vi "Store Static VI References for Subpanel.vi"(8 "error in (no error)":errorcluster, 11 "Controller Configuration in":refnum<class "Controller Configuration.lvclass">) -> (0 "error out":errorcluster, 3 "Controller Configuration out":refnum<class "Controller Configuration.lvclass">)   [LabVIEW 2016, in "Msmt Configuration.lvlib" / "Controller Configuration.lvclass"]
uses:
  Controller Configuration.lvclass
  \\Mac\Home/Documents/Extensible-Config-Dialog/Configuration.lvclass
  Extensible-Config-Dialog/Configuration.lvclass
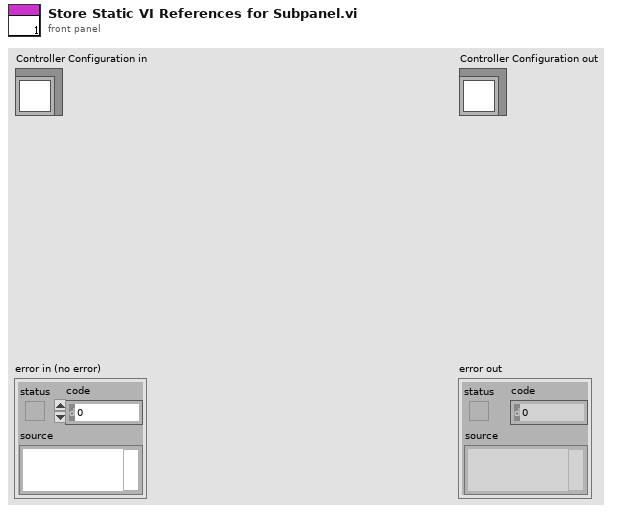
[diagram p1: front panel]
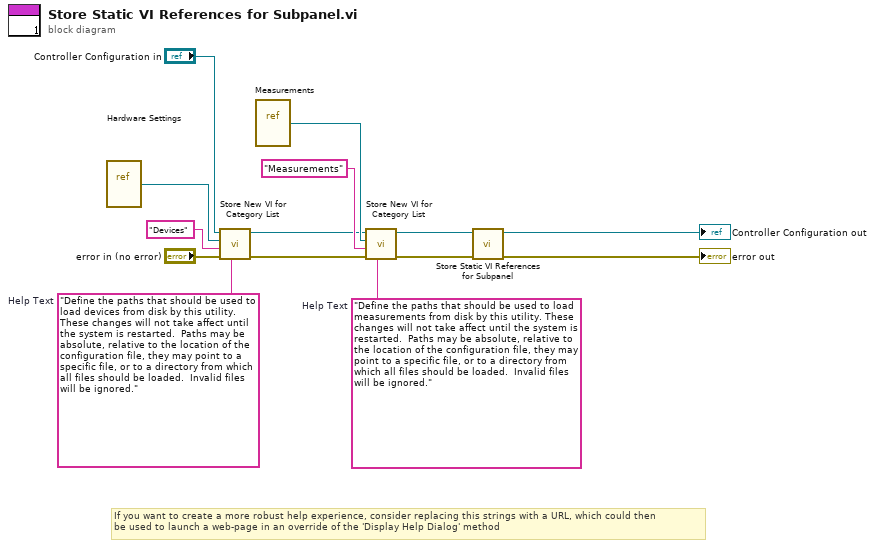
[diagram p0: block diagram]
diagram:
  w1 = "Define the paths that should be used to load devices from disk by this utility. These changes will not take affect until the system is restarted.  Paths may be absolute, relative to the location of the configuration file, they may point to a specific file, or to a directory from which all files should be loaded.  Invalid files will be ignored."  # Help Text
  w2 = "Define the paths that should be used to load measurements from disk by this utility. These changes will not take affect until the system is restarted.  Paths may be absolute, relative to the location of the configuration file, they may point to a specific file, or to a directory from which all files should be loaded.  Invalid files will be ignored."  # Help Text
  # "If you want to create a more robust help experience, consider replacing this strings with a URL, which could then\nbe used to launch a web-page in an override of the 'Display Help Dialog' method"
  n1 = vi-ref "Hardware Settings.vi"() -> (w11:refnum<vi>)
  n2 = call "Store New VI for Category List.vi"("Help Text"=w1, "error in (no error)"="error in (no error)", "String"="Devices", "VI Refnum"=w11, "Configuration in"="Controller Configuration in") -> ("error out"=w7:errorcluster, "Configuration out"=w9:refnum<class "Controller Configuration.lvclass">)  [unwired: 5 in]
  n3 = vi-ref "Measurements.vi"() -> (w13:refnum<vi>)
  n4 = call "Store New VI for Category List.vi"("Help Text"=w2, "error in (no error)"=w7, "String"="Measurements", "VI Refnum"=w13, "Configuration in"=w9) -> ("error out"=w5:errorcluster, "Configuration out"=w4:refnum<class "Controller Configuration.lvclass">)  [unwired: 5 in]
  n5 = call-parent "Store Static VI References for Subpanel.vi"("error in (no error)"=w5, "Configuration in"=w4) -> ("error out"=→"error out":errorcluster, "Configuration out"=→"Controller Configuration out":refnum<class "Controller Configuration.lvclass">)  [unwired: 8 in]
